vi "Write Pattern.vi"(8 "error in (no error)":errorcluster, 9 "IO Lines Pattteen":T1[](array[typedef]) {"Duration (us)" min=0.005 max=42550000.0 step=0.005 format="%#.3f"}, 10 "IO Lines Enable":T2={"Enable"=[FALSE, FALSE, FALSE, FALSE, FALSE, FALSE, FALSE, FALSE, FALSE, FALSE, FALSE, FALSE, FALSE, FALSE, FALSE, FALSE, FALSE, FALSE, FALSE, FALSE, FALSE, FALSE, FALSE, FALSE, FALSE, FALSE, FALSE, FALSE, FALSE, FALSE, FALSE, FALSE]}, 11 "Refnum in":refnum<k20>) -> (0 "error out":errorcluster, 2 "Pattern Digital Data":digitaldata, 3 "FPGA VI Reference Out":refnum<k20>)   [LabVIEW 2016]
uses:
  Typedefs/IO Lines Enable.ctl
  Typedefs/IO Lines State.ctl
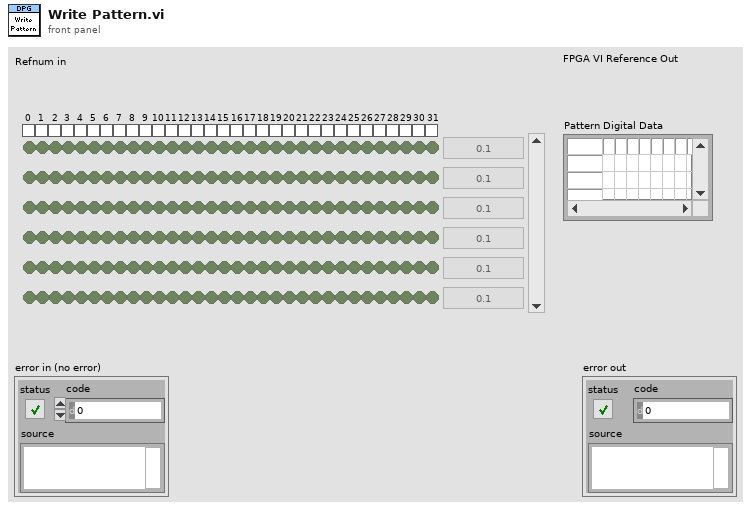
[diagram p1: front panel]
types:
  T1 = typedef "IO Lines State.ctl" = cluster{"State":bool[], "Duration (us)":dbl}
  T2 = typedef "IO Lines Enable.ctl" = cluster{"Enable":bool[]}
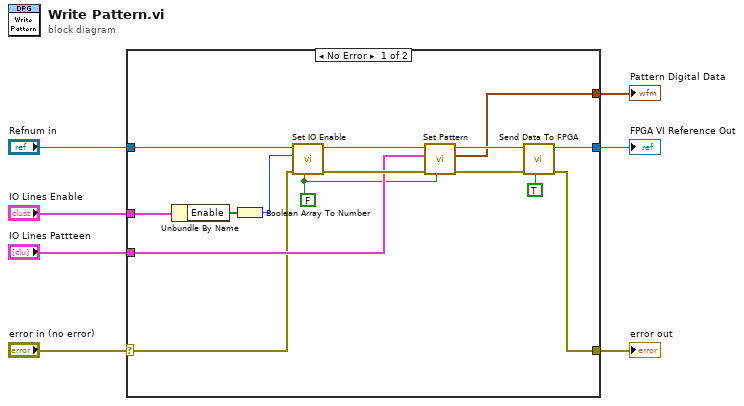
[diagram p0: block diagram]
diagram:
  n1 = case shown="No Error" "error in (no error)" {
    selector: "error in (no error)" -> [w17 w24]
    tunnel: [w13 w24] -> w7
    tunnel: "IO Lines Pattteen" -> [w21 _]
    tunnel: "Refnum in" -> [w14 w23]
    tunnel: "IO Lines Enable" -> [w18 _]
    tunnel: [w8 _] -> w2
    tunnel: [w9 w23] -> w1
    frame No Error {
      w16 = FALSE ("Write to FPGA(T)")
      n2 = Unbundle By Name(w18) -> ("Enable"=w19:bool[])
      n3 = Boolean Array To Number(Boolean array=w19) -> (number=w20:u32)
      n4 = call "Set IO Enable.vi"("Write to FPGA(T)"=w16, "error in (no error)"=w17, "Write Enable"=w20, "FPGA VI Reference In"=w14) -> ("error out"=w22:errorcluster, "FPGA VI Reference Out"=w11:refnum<k20>)  [unwired: 6 in]
      n5 = call "Set Pattern.vi"("Write to FPGA(T)"=w16, "error in (no error)"=w22, "IO Lines Patttern Settings"=w21, "FPGA VI Reference In"=w11) -> ("error out"=w15:errorcluster, "Pattern Digital Data"=w8:digitaldata, "FPGA VI Reference Out"=w10:refnum<k20>)  [unwired: 4 in]
      n6 = call "Send Data To FPGA.vi"("Write to FPGA(T)"=TRUE, "error in (no error)"=w15, "FPGA VI Reference In"=w10) -> ("error out"=w13:errorcluster, "FPGA VI Reference Out"=w9:refnum<k20>)  [unwired: 7 in]
    }
    frame Error {
    }
  }
  "error out" <- w7
  "Pattern Digital Data" <- w2
  "FPGA VI Reference Out" <- w1
